vi "Robot Global Data.vi"() -> ()   [LabVIEW 2019]
doc: "This global VI can contain as many global variables as you need. Place a control on the panel, give it a good name. To read or write to it from a VI, drag the icon to the diagram of that VI. You can also drag from the project. Click on the node to change which global you access. You shouldn't have multiple locations writing to a global or it will cause a race-condition."
uses:
  <vilib>/Rock Robotics/WPI/Camera/WPI_CameraImageSize.ctl
  <vilib>/Rock Robotics/WPI/DriverStation/WPI_DriverStationRobotMode2.ctl
  <vilib>/Rock Robotics/WPI/Solenoid/WPI_SolenoidValue.ctl
panel:
  in  "Climb Motor":dbl
  in  "Vanna":dbl
  in  "Shoot":dbl
  in  "Intake Motor Value":dbl
  in  "Intake Pneumatic Mode":T1
  in  "Auton Values":T2(array[cluster])
  out "Right Drive Sensors":T3
  out "Left Drive Sensors":T4
  in  "Drive Control":enum16{"Driver", "Auton"}(ring)
  in  "Teleop Drive Motor Values":T5
  in  "Robot Mode":T6
  in  "image size":T7=enum."320x240"
  in  "Enable Vision":bool
  # "Please elaborate on this"
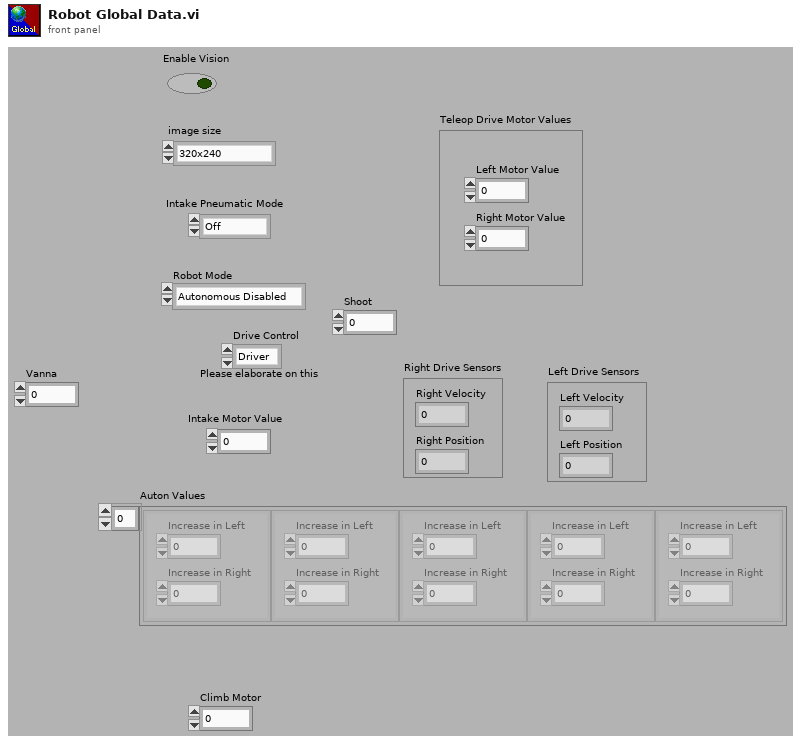
[diagram p1: front panel]
types:
  T1 = typedef "WPI_SolenoidValue.ctl" = enum16{"Off", "On", "Forward", "Reverse"}
  T2 = cluster{"Increase in Left":dbl, "Increase in Right":dbl}[]
  T3 = cluster{"Right Velocity":dbl, "Right Position":dbl}
  T4 = cluster{"Left Velocity":dbl, "Left Position":dbl}
  T5 = cluster{"Left Motor Value":dbl, "Right Motor Value":dbl}
  T6 = typedef "WPI_DriverStationRobotMode2.ctl" = enum16{"Autonomous Disabled", "Autonomous Enabled", "Teleop Disabled", "Teleop Enabled", "Disconnected", "Finish", "Test Disabled", "Test Enabled", "Emergency Stopped"}
  T7 = typedef "WPI_CameraImageSize.ctl" = enum16{"640x480", "320x240", "160x120", "Custom"}
diagram:
